vi "Motion-Move-XandY.vi"(4 "Y Drive Acc/Speed/Velocity":string="MA1: A 10: V 20: AD 10: D ", 6 "X Drive Acc/Speed/Velocity":string="MA1: A 10: V 20: AD 10: D ", 8 "error in (no error)":errorcluster, 9 "X Coordinates":string="-880000", 10 "Y Coordinates":string="880000", 11 "Motion-ControlAll in":refnum<class "Motion-ControlAll.lvclass">) -> (0 "error out":errorcluster, 3 "Motion-ControlAll out":refnum<class "Motion-ControlAll.lvclass">)   [LabVIEW 2013, in "Motion-ControlAll.lvclass"]
uses:
  Motion-ControlAll.lvclass
  Motion-ControlAll.lvclass/Motion-ControlAll.ctl
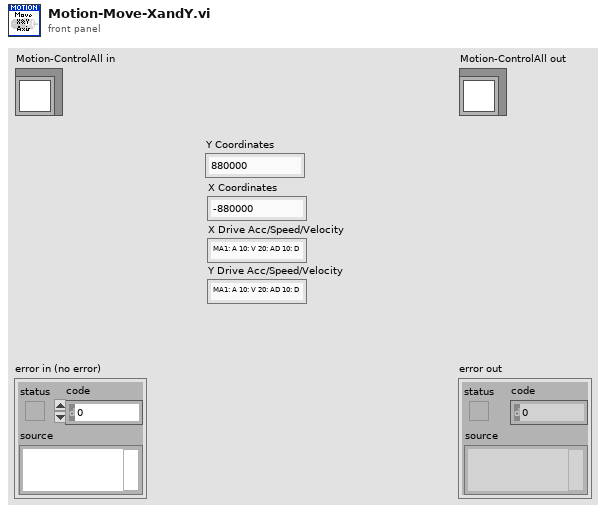
[diagram p1: front panel]
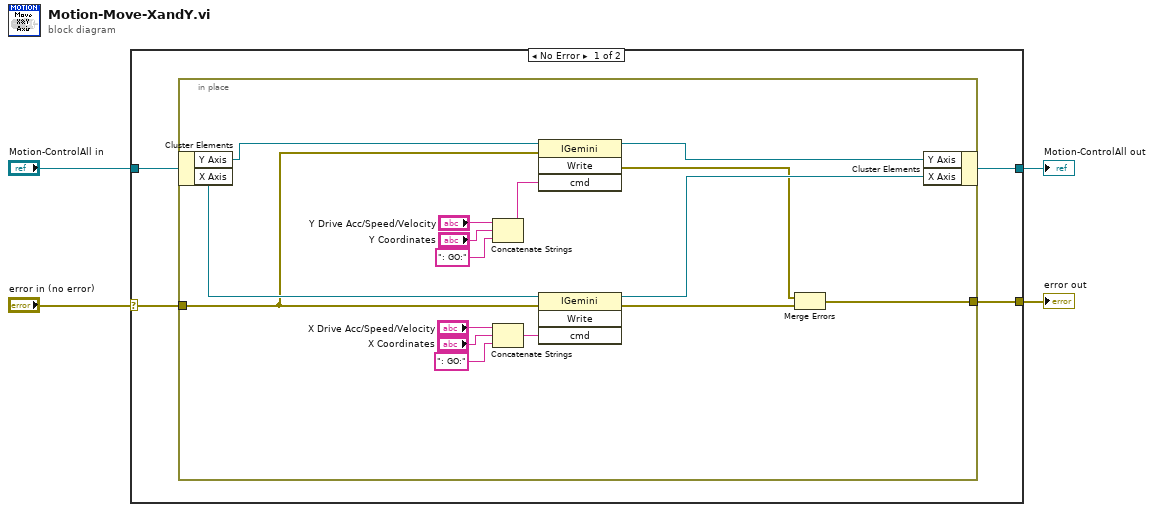
[diagram p0: block diagram]
diagram:
  n1 = case shown="No Error" "error in (no error)" {
    selector: "error in (no error)" -> [w7 w26]
    tunnel: [w6 w26] -> w3
    tunnel: [w5 w25] -> w1
    tunnel: "Motion-ControlAll in" -> [w8 w25]
    frame No Error {
      n2 = in-place {
        in-place-border: w7 -> [w15]
        in-place-border: [w9] -> w6
        n3 = in-place-cluster #1(w8) -> ("Y Axis"=w14:refnum<k7>, "X Axis"=w20:refnum<k7>)
        n4 = Concatenate Strings("Y Drive Acc/Speed/Velocity", "Y Coordinates", ": GO:" ("string")) -> (w19:string)
        n5 = Concatenate Strings("X Drive Acc/Speed/Velocity", "X Coordinates", ": GO:" ("string")) -> (w21:string)
        n6 = invoke class="IGemini" method="Write"(reference=w14, error in=w15, "cmd"=w19) -> (reference out=w13:refnum<k7>, error out=w10:errorcluster)  [unwired: 1 in, 2 out]
        n7 = invoke class="IGemini" method="Write"(reference=w20, error in=w15, "cmd"=w21) -> (reference out=w12:refnum<k7>, error out=w11:errorcluster)  [unwired: 1 in, 2 out]
        n8 = Merge Errors(w10, w11) -> (w9:errorcluster)
        n9 = in-place-cluster #1("Y Axis"=w13, "X Axis"=w12) -> (w5:refnum<class "Motion-ControlAll.lvclass">)
      }
    }
    frame Error {
    }
  }
  "error out" <- w3
  "Motion-ControlAll out" <- w1
